vi "dash safety data FG.vi"(1 "Safety Data":T1, 2 "Menu":T2) -> (0 "Safety Data Out":T1)   [LabVIEW 2013]
uses:
  typedefs/fg_typedef.ctl
  typedefs/dashboard safety status data.ctl
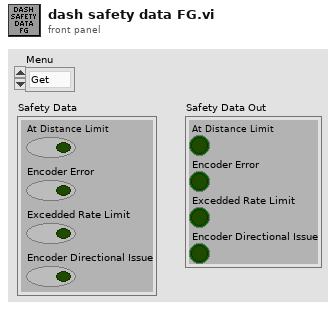
[diagram p1: front panel]
types:
  T1 = typedef "dashboard safety status data.ctl" = cluster{"At Distance Limit":bool, "Encoder Error":bool, "Excedded Rate Limit":bool, "Encoder Directional Issue":bool}
  T2 = typedef "fg_typedef.ctl" = enum16{"Get", "Set"}
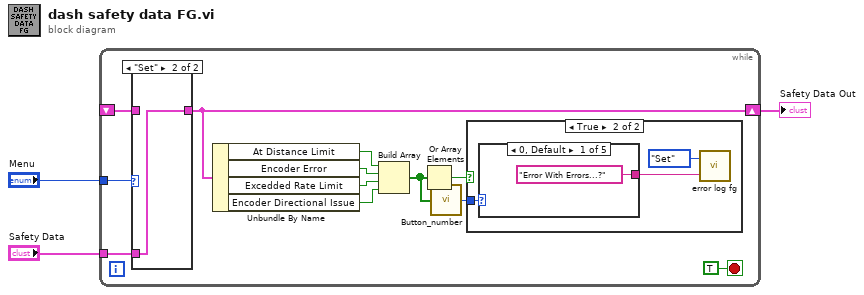
[diagram p0: block diagram]
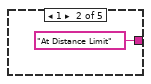
[diagram p3: hidden frame]
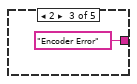
[diagram p4: hidden frame]
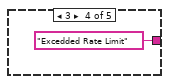
[diagram p5: hidden frame]
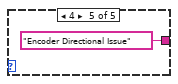
[diagram p6: hidden frame]
diagram:
  n1 = while {
    tunnel: "Menu" -> [w14]
    shift-right: [w11] -> w1
    shift-left: _ -> [w13]
    tunnel: "Safety Data" -> [w12]
    stop <- TRUE stop-if-true
    n2 = case shown="\"Set\"" w14 {
      tunnel: w13 -> [w24 _]
      tunnel: [w24 w25] -> w11
      tunnel: w12 -> [_ w25]
      frame "Get", Default {
      }
      frame "Set" {
      }
    }
    n3 = Unbundle By Name(w11) -> ("At Distance Limit"=w10:bool, "Encoder Error"=w9:bool, "Excedded Rate Limit"=w8:bool, "Encoder Directional Issue"=w7:bool)
    n4 = Build Array(w10, w9, w8, w7) -> (w5:bool[])
    n5 = Or Array Elements(Boolean array=w5) -> (logical OR=w6:bool)
    n6 = call "Button_number.vi"("Button Array"=w5) -> ("Button Pressed"=w4:i32)
    n7 = case shown="True" w6 {
      tunnel: w4 -> [_ w17]
      frame False {
      }
      frame True {
        n8 = case shown="0, Default" w17 {
          tunnel: ["Error With Errors...?" "At Distance Limit" "Encoder Error" "Excedded Rate Limit" "Encoder Directional Issue"] -> w16
          frame 0, Default {
          }
          frame 1 {
          }
          frame 2 {
          }
          frame 3 {
          }
          frame 4 {
          }
        }
        n9 = call "error log fg.vi"("Error"=w16, "Log Mode"=enum16{"Get", "Set", "Clear"}."Set") -> ()  [unwired: 2 out]
      }
    }
  }
  "Safety Data Out" <- w1
